vi "GenerateIndexedPath.vi"(6 "number":i32, 9 "stop":dbl, 10 "start":dbl, 11 "input folder":path) -> (3 "output path":path)   [LabVIEW 2018]
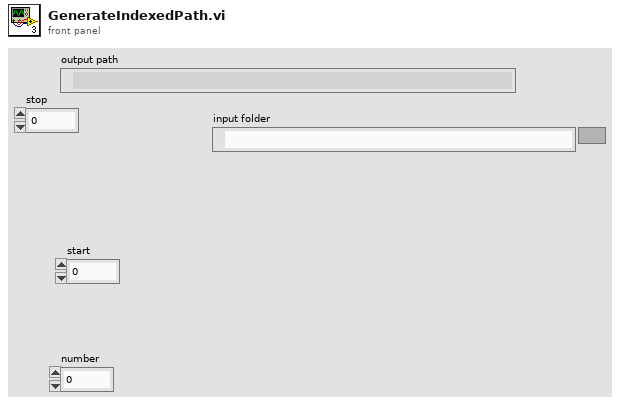
[diagram p1: front panel]
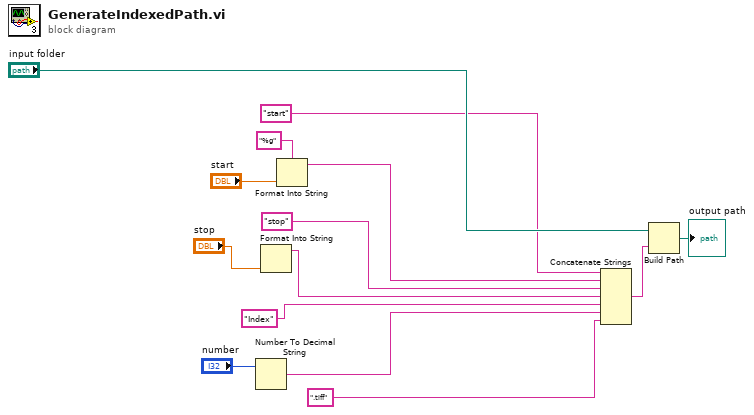
[diagram p0: block diagram]
diagram:
  n1 = Number To Decimal String(number="number") -> (decimal integer string=w7:string)  [unwired: 1 in]
  n2 = Format Into String("stop") -> (resulting string=w1:string)  [unwired: 3 in, 1 out]
  n3 = Format Into String(format string="%g", "start") -> (resulting string=w4:string)  [unwired: 2 in, 1 out]
  n4 = Concatenate Strings("start" ("name or relative path"), w4, "stop" ("name or relative path"), w1, "Index" ("name or relative path"), w7, ".tiff" ("name or relative path")) -> (w11:string)
  n5 = Build Path(base path="input folder", name or relative path=w11) -> (appended path=→"output path":path)
